vi "Generate config File.vi"(8 "error in (no error)":errorcluster, 10 "Path to top-level Directory":path, 11 "Path to generated ini file":path) -> (0 "error out":errorcluster)   [LabVIEW 2026]
uses:
  Hardware Paths Cluster.ctl
  Measurement Paths Cluster.ctl
  MAL-Framework/user.lib/Common Components/Measurement Actor/Measurement.lvclass
  MAL-Framework/user.lib/Common Components/Hardware/Hardware.lvclass
  <userlib>/_OpenG.lib/file/file.llb/Compare Two Paths - Scalar__ogtk.vi
  recovery/packages/oglib_file-4.0.1.22-8A89CE420A/File Group 0/user.lib/_OpenG.lib/file/file.llb/Build Path - Traditional - path__ogtk.vi
  <vilib>/Utility/config.llb/Write Key (Boolean).vi
  <vilib>/Utility/config.llb/NI_LVConfig.lvlib
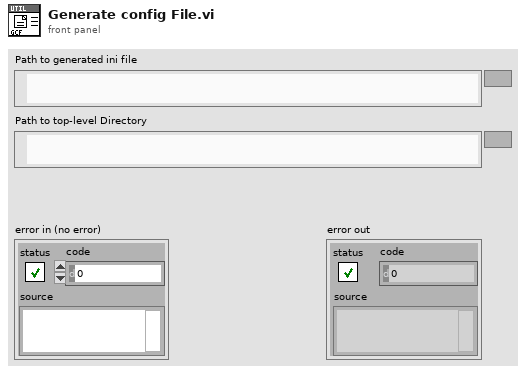
[diagram p1: front panel]
types:
  T1 = typedef "Measurement Paths Cluster.ctl" = cluster{"Paths":path[]}
  T2 = typedef "Hardware Paths Cluster.ctl" = cluster{"Paths":path[]}
  T3 = typedef "NI_LVConfig.lvlib/Config Data RefNum.ctl" = refnum<k1>
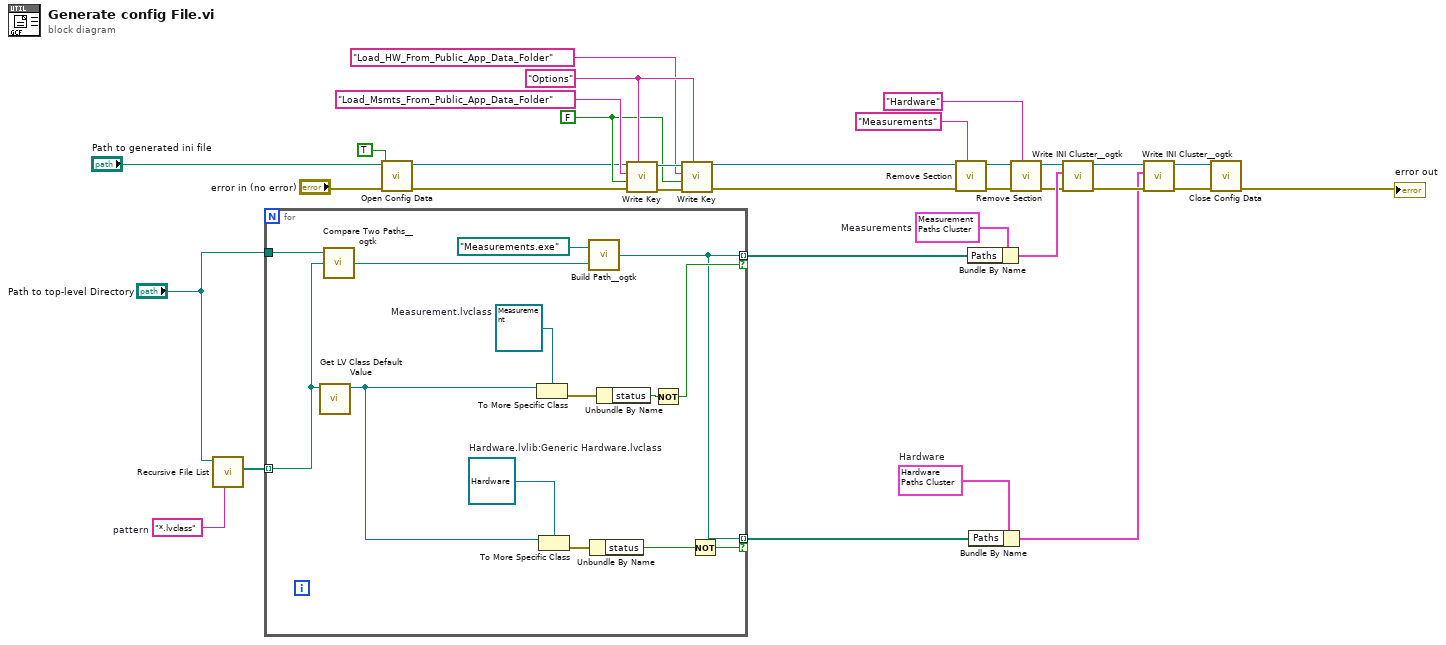
[diagram p0: block diagram]
diagram:
  w6 = FALSE ("value")
  w7 = "Options" ("section")
  w23 = T1 {"Paths"=[path "C:/Users/ekerry/Projects/Measurement Utility/Source/Framework/Measurements"]}  # Measurements
  w22 = T2 {"Paths"=[path "C:/Users/ekerry/Projects/Measurement Utility/Source/Framework/Installed Hardware"]}  # Hardware
  w31 = "*.lvclass"  # pattern
  n1 = call <vilib>:"Recursive File List.vi"("pattern"=w31, "Folder Path"="Path to top-level Directory") -> ("All Files in Dir"=w32:path[])  [unwired: 5 in, 4 out]
  n2 = for {
    tunnel: w32 -> [w44] mode=indexing
    tunnel: "Path to top-level Directory" -> [w46]
    tunnel: [w35] -> w19 mode=indexing if=w38
    tunnel: [w35] -> w18 mode=indexing if=w39
    w34 = refnum<class "Hardware.lvclass"> refnum  # Hardware.lvlib:Generic Hardware.lvclass
    w45 = refnum<class "Measurement.lvclass"> refnum  # Measurement.lvclass
    n3 = call <vilib>:"Get LV Class Default Value.vi"("class path"=w44) -> ("object"=w47:refnum<class>)  [unwired: 9 in, 1 out]
    n4 = call-poly <userlib>:"Compare Two Paths__ogtk.vi"("path2"=w44, "path1"=w46) -> ("relative path from 1 to 2"=w37:path)  [unwired: 1 in, 2 out]
    n5 = To More Specific Class(target class=w45, reference=w47) -> (error out=w43:errorcluster)  [unwired: 1 in, 1 out]
    n6 = To More Specific Class(target class=w34, reference=w47) -> (error out=w42:errorcluster)  [unwired: 1 in, 1 out]
    n7 = call-poly "Build Path__ogtk.vi"("name or relative path"=w37, "base path"=path "Measurements.exe") -> ("appended path"=w35:path)
    n8 = Unbundle By Name(w42) -> ("status"=w41:bool)
    n9 = Unbundle By Name(w43) -> ("status"=w40:bool)
    n10 = Not(x=w40) -> (.not. x?=w39:bool)
    n11 = Not(x=w41) -> (.not. x?=w38:bool)
  }
  n12 = call <vilib>:"Open Config Data.vi"("error in (no error)"="error in (no error)", "create file if necessary (T)"=TRUE, "configuration file path"="Path to generated ini file") -> ("error out"=w1:errorcluster, "refnum"=w4:T3)  [unwired: 6 in, 1 out]
  n13 = call-poly <vilib>:"Write Key.vi"("section"=w7, "error in (no error)"=w1, "value"=w6, "key"="Load_Msmts_From_Public_App_Data_Folder", "refnum"=w4) -> ("error out"=w10:errorcluster, "refnum out"=w9:T3)  [unwired: 4 in, 1 out]
  n14 = call-poly <vilib>:"Write Key.vi"("section"=w7, "error in (no error)"=w10, "value"=w6, "key"="Load_HW_From_Public_App_Data_Folder", "refnum"=w9) -> ("error out"=w2:errorcluster, "refnum out"=w3:T3)  [unwired: 4 in, 1 out]
  n15 = call <vilib>:"Remove Section.vi"("section"="Measurements" ("float number format (optional)"), "error in (no error)"=w2, "refnum"=w3) -> ("error out"=w12:errorcluster, "refnum out"=w16:T3)  [unwired: 6 in, 1 out]
  n16 = Bundle By Name(cluster=w23, "Paths"=w18) -> (w20:T1)
  n17 = Bundle By Name(cluster=w22, "Paths"=w19) -> (w21:T2)
  n18 = call <vilib>:"Remove Section.vi"("section"="Hardware" ("float number format (optional)"), "error in (no error)"=w12, "refnum"=w16) -> ("error out"=w11:errorcluster, "refnum out"=w14:T3)  [unwired: 6 in, 1 out]
  n19 = call <userlib>:"Write INI Cluster__ogtk.vi"("error in (no error)"=w11, "INI Fomatted Cluster"=w20, "refnum"=w14) -> ("error out"=w25:errorcluster, "dup refnum"=w24:T3)  [unwired: 7 in]
  n20 = call <userlib>:"Write INI Cluster__ogtk.vi"("error in (no error)"=w25, "INI Fomatted Cluster"=w21, "refnum"=w24) -> ("error out"=w27:errorcluster, "dup refnum"=w26:T3)  [unwired: 7 in]
  n21 = call <vilib>:"Close Config Data.vi"("error in (no error)"=w27, "refnum"=w26) -> ("error out"=→"error out":errorcluster)  [unwired: 8 in, 1 out]
